vi "angle to encoder.vi"(9 "red angle":dbl, 10 "blue angle":dbl) -> (1 "red encoder":dbl, 2 "blue encoder":dbl)   [LabVIEW 2020]
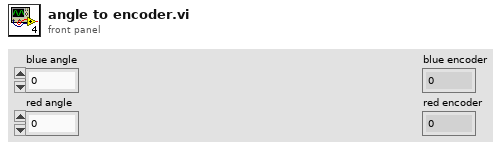
[diagram p1: front panel]
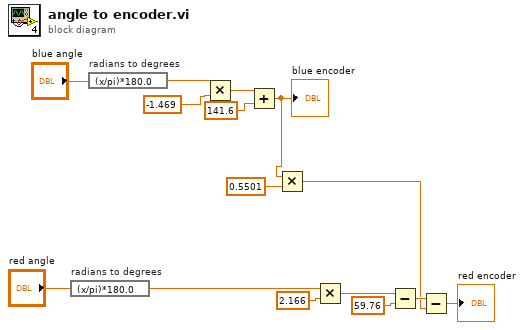
[diagram p0: block diagram]
diagram:
  n1 = expression code="(x/pi)*180.0" "radians to degrees"("red angle") -> (w1:dbl)
  n2 = expression code="(x/pi)*180.0" "radians to degrees"("blue angle") -> (w2:dbl)
  n3 = Multiply(x=w2, y=-1.469) -> (x*y=w12:dbl)
  n4 = Add(x=w12, y=141.6) -> (x+y=w7:dbl)
  "blue encoder" <- w7
  n5 = Multiply(x=w7, y=0.5501) -> (x*y=w4:dbl)
  n6 = Multiply(x=w1, y=2.166) -> (x*y=w9:dbl)
  n7 = Subtract(x=w9, y=59.76) -> (x-y=w5:dbl)
  n8 = Subtract(x=w5, y=w4) -> (x-y=→"red encoder":dbl)
